vi "AH_msgTEST.vi"() -> ()   [LabVIEW 2021]
uses:
  Data_Cluster.ctl
  Measurement_Cluster.ctl
  Config_Cluster.ctl
  Mode_Enum.ctl
  AH_CmdSRE.vi
panel:
  in  "Configuration Cluster":T1={"General"={"Config.ini"=path "", "Default Logging Path"=path ""}, "Hardware"={"AHC VISA COM"="", "Measure Rate (1/s)"=0, "Global T VAR"="", "Global B VAR"=""}, "Operation"={"Operation Mode"=enum."Idle-Off", "Status"="", "NewLog?"=FALSE}}
  in  "Data Cluster In":T3 {"GUI Data Cluster"."SBR" format="%08b"}
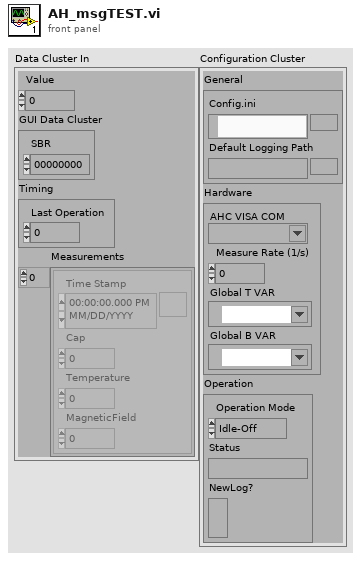
[diagram p1: front panel]
types:
  T1 = typedef "Config_Cluster.ctl" = cluster{"General":cluster{"Config.ini":path, "Default Logging Path":path}, "Hardware":cluster{"AHC VISA COM":refnum<visa-resource-name>, "Measure Rate (1/s)":i32, "Global T VAR":refnum<k21>, "Global B VAR":refnum<k21>}, "Operation":cluster{"Operation Mode":T2, "Status":string, "NewLog?":bool}}
  T2 = typedef "Mode_Enum.ctl" = enum16{"Logging", "Idle-Off", "Idle"}
  T3 = typedef "Data_Cluster.ctl" = cluster{"Value":dbl, "GUI Data Cluster":cluster{"SBR":u16}, "Timing":cluster{"Last Operation":dbl}, "Measurements":T4[]}
  T4 = typedef "Measurement_Cluster.ctl" = cluster{"Time Stamp":timestamp, "Cap":dbl, "Temperature":dbl, "MagneticField":dbl}
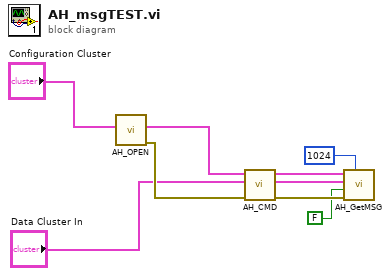
[diagram p0: block diagram]
diagram:
  n1 = call "AH_OPEN.vi"("Configuration Cluster"="Configuration Cluster") -> ("error out"=w8:errorcluster, "Configuration Cluster Out"=w9:T1)  [unwired: 9 in]
  n2 = call-poly "AH_CMD.vi"("error in (no error)"=w8, "Data Cluster In"="Data Cluster In", "Config Cluster In"=w9) -> ("error IO"=w3:errorcluster, "Data Cluster Out"=w4:T3, "Configuration Cluster Out"=w5:T1)  [unwired: 6 in]
  n3 = call "AH_GetMSG.vi"("byte count"=u32 1024, "error in (no error)"=w3, "Halt For RQS"=FALSE, "Data Cluster In"=w4, "Config Cluster In"=w5) -> ()  [unwired: 1 in, 6 out]
